vi "_FlattenStrPtr To HexStrPtr.vi"(1 "FlattenStrPtr":string) -> (0 "HexStrPtr":string)   [LabVIEW 2014]
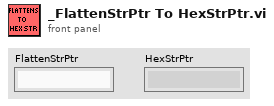
[diagram p1: front panel]
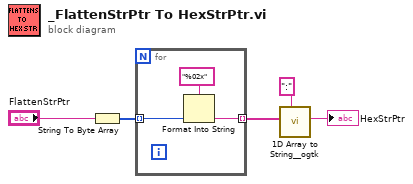
[diagram p0: block diagram]
diagram:
  n1 = String To Byte Array(string="FlattenStrPtr") -> (unsigned byte array=w2:u8[])
  n2 = for {
    tunnel: [w7] -> w4 mode=indexing
    tunnel: w2 -> [w8] mode=indexing
    n3 = Format Into String(format string="%02x", w8) -> (resulting string=w7:string)  [unwired: 2 in, 1 out]
  }
  n4 = call <userlib>:"1D Array to String__ogtk.vi"("delimiter (Tab)"=":", "Array of Strings"=w4) -> ("delimited string"=→"HexStrPtr":string)  [unwired: 9 in]
